vi "Configure.vi"(8 "error in":errorcluster, 10 "Output Settings":T1={"Voltage (V)"=1.0} {"Voltage (V)" min=-424.2 max=424.2 step=1.0 format="%#.1f"}, 11 "UDP in":refnum<class "UDP.lvclass">) -> (0 "error out":errorcluster, 3 "UDP out":refnum<class "UDP.lvclass">)   [LabVIEW 2020, in "Plugin Instrument Driver.lvlib" / "UDP.lvclass"]
doc: "Sets the output channel"
uses:
  UDP.lvclass
  Typedefs/Output Settings.ctl
  Typedefs/Device Details.ctl
  Instrument Driver.lvclass
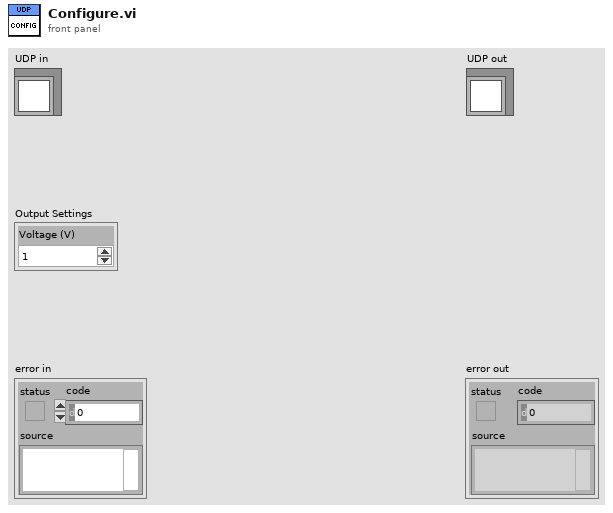
[diagram p1: front panel]
types:
  T1 = typedef "Plugin Instrument Driver.lvlib/Instrument Driver.lvclass/Output Settings.ctl" = cluster{"Voltage (V)":dbl}
  T2 = typedef "Plugin Instrument Driver.lvlib/UDP.lvclass/Device Details.ctl" = cluster{"Device Port Number":u16, "Device IP":string, "Timeout":i32, "Port Number":u16, "Connection ID":refnum<k16>}
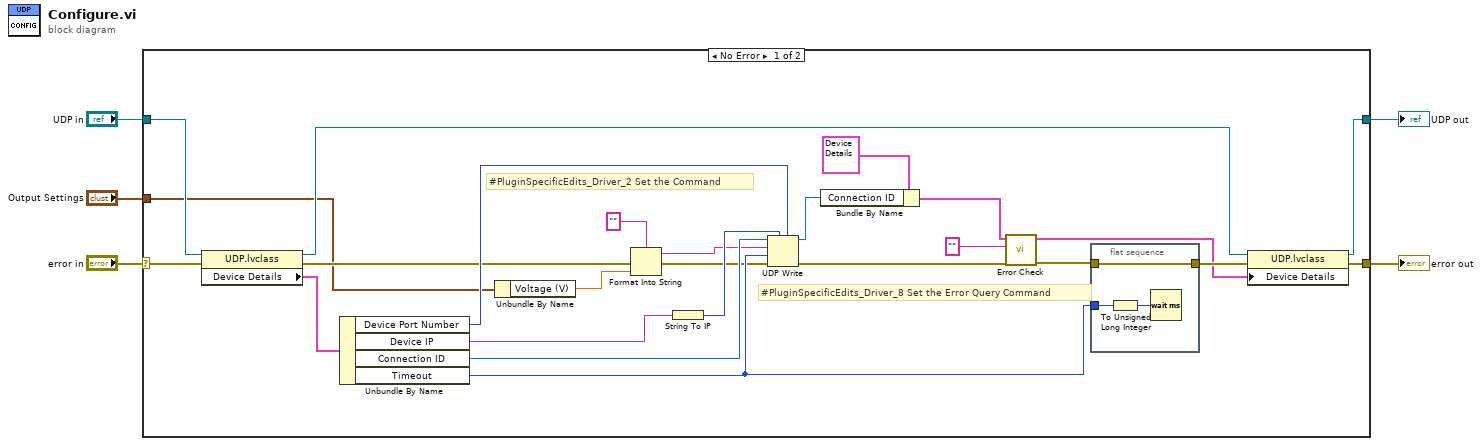
[diagram p0: block diagram]
diagram:
  n1 = case shown="No Error" "error in" {
    selector: "error in" -> [w29 w35]
    tunnel: "UDP in" -> [w28 w34]
    tunnel: [w24 w35] -> w3
    tunnel: [w25 w34] -> w2
    tunnel: "Output Settings" -> [w10 _]
    frame No Error {
      # "#PluginSpecificEdits_Driver_8 Set the Error Query Command"
      # "#PluginSpecificEdits_Driver_2 Set the Command"
      n2 = property class="UDP.lvclass"(reference=w28, error in=w29) -> (reference out=w27:refnum<class "UDP.lvclass">, error out=w12:errorcluster, "Device Details"=w21:T2)
      n3 = Unbundle By Name(w21) -> ("Device Port Number"=w20:u16, "Device IP"=w19:string, "Connection ID"=w18:refnum<k16>, "Timeout"=w17:i32)
      n4 = Unbundle By Name(w10) -> ("Voltage (V)"=w15:dbl)
      n5 = Format Into String(format string="", error in=w12, w15) -> (resulting string=w13:string, error out=w11:errorcluster)  [unwired: 1 in]
      n6 = String To IP(1:w19) -> (0:w30:u32)
      n7 = UDP Write(address=w30, port or service name=w20, connection ID=w18, data in=w13, 8:w11, 9:w17) -> (error out=w23:errorcluster, 3:w8:refnum<k16>)
      n8 = Bundle By Name(cluster=T2 {"Device Port Number"=2001, "Device IP"="192.168.1.1.100", "Timeout"=5000, "Port Number"=1234, "Connection ID"=refnum} ("Device Details"), "Connection ID"=w8) -> (w7:T2)
      n9 = call "Error Check.vi"("error in"=w23, "Error Query Command"="" ("data in"), "Device Details in"=w7) -> ("error out"=w22:errorcluster, "Device Details out"=w6:T2)  [unwired: 7 in]
      n10 = flat-sequence {
        tunnel: [w31] -> w26
        tunnel: w22 -> [w31]
        tunnel: w17 -> [w33]
        frame #0 {
          n11 = To Unsigned Long Integer(number=w33) -> (unsigned 32bit integer=w32:u32)
          n12 = Wait (ms)(milliseconds to wait=w32) -> ()  [unwired: 1 out]
        }
      }
      n13 = property class="UDP.lvclass"(reference=w27, error in=w26, "Device Details"=w6) -> (reference out=w25:refnum<class "UDP.lvclass">, error out=w24:errorcluster)
    }
    frame Error {
    }
  }
  "error out" <- w3
  "UDP out" <- w2
